vi "vi call by reference.vi"() -> ()   [LabVIEW 2019]
panel:
  in  "X":dbl
  in  "Y":dbl
  out "x+y":dbl
  out "error out":errorcluster
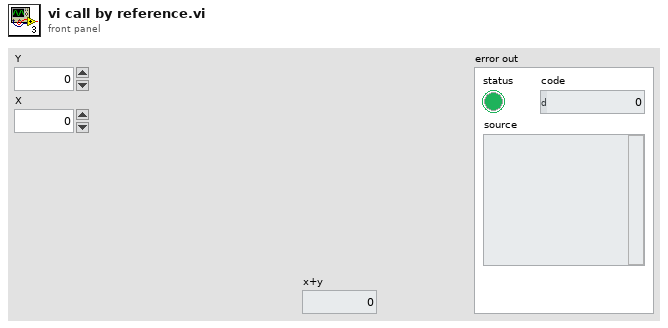
[diagram p1: front panel]
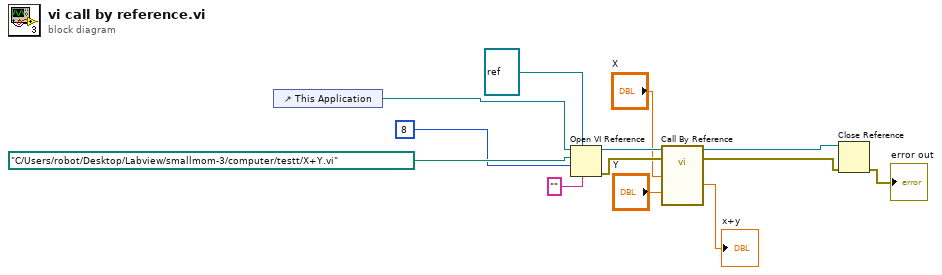
[diagram p0: block diagram]
diagram:
  n1 = control-ref of="This Application"() -> (w1:refnum<vi>)
  n2 = Open VI Reference(type specifier VI Refnum (for type only)=refnum<vi> refnum ("application reference (local)"), application reference (local)=w1, vi path=path "C:/Users/robot/Desktop/Labview/smallmom-3/computer/testt/X+Y.vi", options=8, password ("")="") -> (vi reference=w10:refnum<vi>, error out=w9:errorcluster)  [unwired: 1 in]
  n3 = call-by-ref "?"(reference=w10, error in=w9, "Y"="Y", "X"="X") -> (reference out=w8:refnum<vi>, error out=w7:errorcluster, "x+y"=→"x+y":dbl)
  n4 = Close Reference(reference=w8, error in (no error)=w7) -> (error out=→"error out":errorcluster)
